vi "Get Base Protocol.vi"(8 "error in (no error)":errorcluster, 11 "Protocol Parent in":refnum<class "Protocol Parent.lvclass">) -> (0 "error out":errorcluster, 2 "Protocol out":T1, 3 "Protocol Parent out":refnum<class "Protocol Parent.lvclass">)   [LabVIEW 2013, in "Protocol Classes.lvlib" / "Protocol Parent.lvclass"]
uses:
  Protocol Parent.lvclass
  Types/Base Protocol Type.ctl
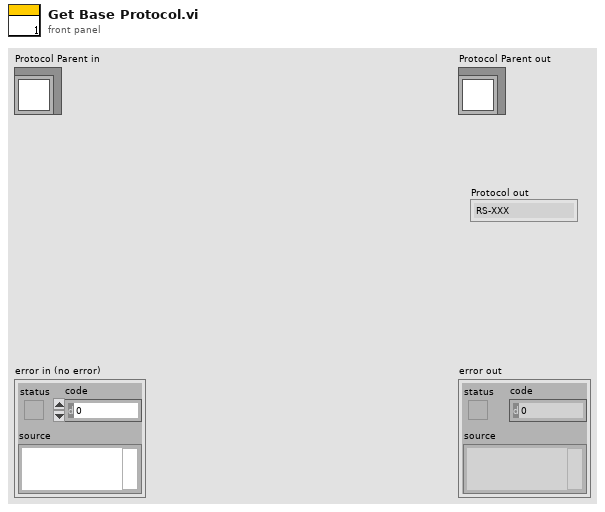
[diagram p1: front panel]
types:
  T1 = typedef "Protocol Classes.lvlib/Protocol Parent.lvclass/Base Protocol Type.ctl" = enum16{"RS-XXX", "VISA", "TCPIP", "UDP"}
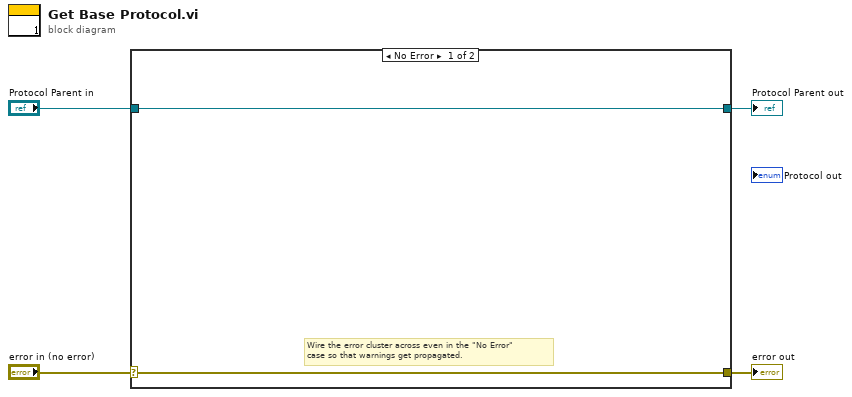
[diagram p0: block diagram]
diagram:
  n1 = case shown="No Error" "error in (no error)" {
    selector: "error in (no error)" -> [w5 w8]
    tunnel: [w5 w8] -> w3
    tunnel: [w6 w7] -> w1
    tunnel: "Protocol Parent in" -> [w6 w7]
    frame No Error {
      # "Wire the error cluster across even in the \"No Error\"\ncase so that warnings get propagated."
    }
    frame Error {
    }
  }
  "error out" <- w3
  "Protocol Parent out" <- w1
